vi "InterfaceExample.vi"() -> ()   [LabVIEW 2017]
uses:
  Interface/Configuration.ctl
  <instrlib>/_niInstr/FIFO Register Bus/v1/Host/niInstr FIFO Register Bus v1 Host.lvclass
  C:/Program Files (x86)/National Instruments/LabVIEW 2017/instr.lib/_niInstr/Instruction Framework/v1/Host/Instruction Target/niInstr Instruction Target v1 Host.lvclass
  <vilib>/FPGAPlugInAG/sbRIO-9607/niLvFpga_Open_sbRIO-9607.vi
  <vilib>/rvi/interface/common/dynamic/niFpgaDynamicAddResources.vi
  <vilib>/Utility/error.llb/Error Cluster From Error Code.vi
  <vilib>/rvi/errors/niLvFpgaAdjustHostInterfaceError.vi
  <vilib>/FPGAPlugInAG/Dynamic/niLvFpga_Close_Dynamic.vi
  <vilib>/rvi/interface/nirviOpenFPGA/nirviOpenFPGA.xnode
  FPGA Bitfiles/ScaleAndLimit_FPGATarget_BasicExampleWith_nkdyZl4UhlU.lvbitx
  <vilib>/rvi/interface/nirviReadWriteControl/nirviReadWriteControl.xnode
  <vilib>/rvi/interface/nirviCloseFPGA/nirviCloseFPGA.xnode
  Interface/ScaleAndLimitInterface.lvlib
  <instrlib>/_niInstr/Instruction Framework/v1/Host/Subsystem Map/niInstr Subsystem Map v1 Host.lvclass
  NiFpgaLv.dll
  <vilib>/rvi/interface/Simulation/niFpgaSimulationCallBeginRW.vi
panel:
  out "ScaledAI":sgl[](array[numeric])
  out "SimultaneousAILoopRate":u32
  in  "DummyChannel15":i16
  in  "stop":bool
  out "Limits":string
  in  "clearLimits":bool
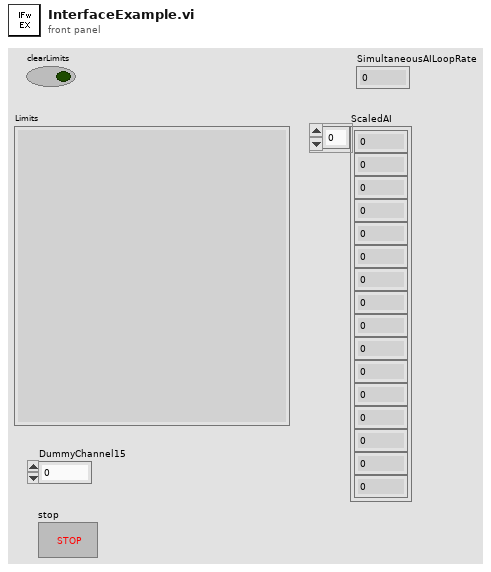
[diagram p1: front panel]
types:
  T1 = typedef "ScaleAndLimitInterface.lvlib/Configuration.ctl" = cluster{"Name":string, "M":dbl, "B":i16, "HighLimit":dbl, "LowLimit":dbl, "LimitsEnabled":bool}
  T2 = typedef "ScaleAndLimitInterface.lvlib/Interface.ctl" = cluster{"instruction target":refnum<class "niInstr Instruction Target v1 Host.lvclass">, "ScalingAndLimitsContext":refnum<class "niInstr Instruction Framework Context v1 Host.lvclass">, "Configuration":T1[]}
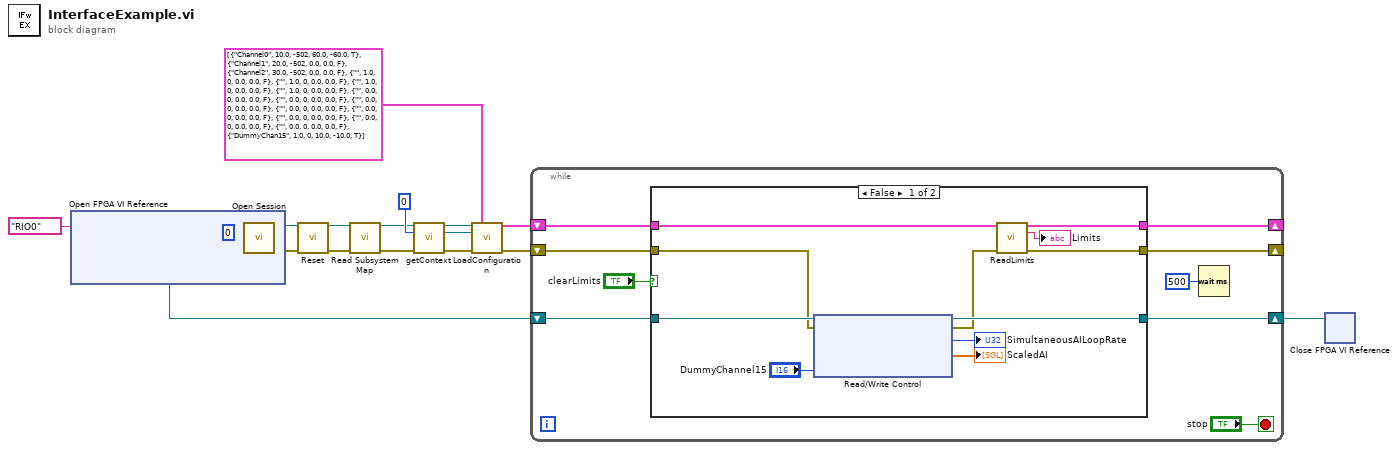
[diagram p0: block diagram]
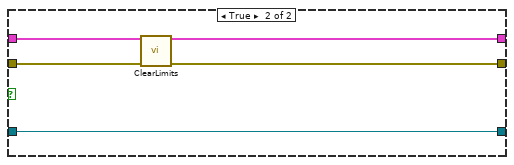
[diagram p2: hidden frame]
diagram:
  n1 = xnode "Open FPGA VI Reference"("resource name"=tag "RIO0") -> ("FPGA VI Reference Out"=w7:refnum<k20>, "error out"=w6:errorcluster)  [unwired: 1 in]
  n2 = call <instrlib>:"Open Session.vi"("fpga ref"=w7, "bus instance"=u32 0, "error in"=w6) -> ("session out"=w10:refnum<class "niInstr FIFO Register Bus v1 Host.lvclass">, "error out"=w11:errorcluster)  [unwired: 11 in]
  n3 = call-dynamic "Reset.vi"("session in"=w10, "error in"=w11) -> ("session out"=w8:refnum<class "niInstr FIFO Register Bus v1 Host.lvclass">, "error out"=w9:errorcluster)  [unwired: 12 in]
  n4 = call <instrlib>:"Read Subsystem Map.vi"("instruction target in"=w8, "error in"=w9) -> ("instruction target out"=w3:refnum<class "niInstr FIFO Register Bus v1 Host.lvclass">, "error out"=w5:errorcluster)  [unwired: 11 in, 1 out]
  n5 = call "getContext.vi"("session in"=w3, "instance"=u8 0, "error in"=w5) -> ("session out"=w2:refnum<class "niInstr FIFO Register Bus v1 Host.lvclass">, "ScalingAndLimitsContext"=w1:refnum<class "niInstr Instruction Framework Context v1 Host.lvclass">, "error out"=w17:errorcluster)  [unwired: 10 in]
  n6 = call "LoadConfiguration.vi"("instruction target in"=w2, "Configuration"=T1[] [{"Name"="Channel0", "M"=10.0, "B"=-502, "HighLimit"=60.0, "LowLimit"=-60.0, "LimitsEnabled"=TRUE}, {"Name"="Channel1", "M"=20.0, "B"=-502, "HighLimit"=0.0, "LowLimit"=0.0, "LimitsEnabled"=FALSE}, {"Name"="Channel2", "M"=30.0, "B"=-502, "HighLimit"=0.0, "LowLimit"=0.0, "LimitsEnabled"=FALSE}, {"Name"="", "M"=1.0, "B"=0, "HighLimit"=0.0, "LowLimit"=0.0, "LimitsEnabled"=FALSE}, {"Name"="", "M"=1.0, "B"=0, "HighLimit"=0.0, "LowLimit"=0.0, "LimitsEnabled"=FALSE}, {"Name"="", "M"=1.0, "B"=0, "HighLimit"=0.0, "LowLimit"=0.0, "LimitsEnabled"=FALSE}, {"Name"="", "M"=1.0, "B"=0, "HighLimit"=0.0, "LowLimit"=0.0, "LimitsEnabled"=FALSE}, {"Name"="", "M"=0.0, "B"=0, "HighLimit"=0.0, "LowLimit"=0.0, "LimitsEnabled"=FALSE}, {"Name"="", "M"=0.0, "B"=0, "HighLimit"=0.0, "LowLimit"=0.0, "LimitsEnabled"=FALSE}, {"Name"="", "M"=0.0, "B"=0, "HighLimit"=0.0, "LowLimit"=0.0, "LimitsEnabled"=FALSE}, {"Name"="", "M"=0.0, "B"=0, "HighLimit"=0.0, "LowLimit"=0.0, "LimitsEnabled"=FALSE}, {"Name"="", "M"=0.0, "B"=0, "HighLimit"=0.0, "LowLimit"=0.0, "LimitsEnabled"=FALSE}, {"Name"="", "M"=0.0, "B"=0, "HighLimit"=0.0, "LowLimit"=0.0, "LimitsEnabled"=FALSE}, {"Name"="", "M"=0.0, "B"=0, "HighLimit"=0.0, "LowLimit"=0.0, "LimitsEnabled"=FALSE}, {"Name"="", "M"=0.0, "B"=0, "HighLimit"=0.0, "LowLimit"=0.0, "LimitsEnabled"=FALSE}, {"Name"="DummyChan15", "M"=1.0, "B"=0, "HighLimit"=10.0, "LowLimit"=-10.0, "LimitsEnabled"=TRUE}], "ScalingAndLimitsContext"=w1, "error in (no error)"=w17) -> ("Interface"=w14:T2, "error out"=w13:errorcluster)  [unwired: 10 in]
  n7 = while {
    shift-right: [w20] -> _
    shift-left: w14 -> [w27]
    shift-right: [w19] -> _
    shift-left: w13 -> [w26]
    shift-right: [w21] -> w12
    shift-left: w7 -> [w22]
    stop <- "stop" stop-if-true
    n8 = case shown="False" "clearLimits" {
      tunnel: w27 -> [w34 w43]
      tunnel: w26 -> [w36 w42]
      tunnel: [w33 w41] -> w20
      tunnel: [w32 w40] -> w19
      tunnel: w22 -> [w38 w39]
      tunnel: [w35 w39] -> w21
      frame False {
        n9 = xnode "Read/Write Control"("FPGA VI Reference In"=w38, "error in"=w36, "DummyChannel15"="DummyChannel15") -> ("FPGA VI Reference Out"=w35:refnum<k20>, "error out"=w30:errorcluster, "SimultaneousAILoopRate"=→"SimultaneousAILoopRate":u32, "ScaledAI"=→"ScaledAI":sgl[])
        n10 = call "ReadLimits.vi"("Interface in"=w34, "error in (no error)"=w30) -> ("Interface out"=w33:T2, "Limits"=→"Limits":string, "error out"=w32:errorcluster)  [unwired: 11 in]
      }
      frame True {
        n11 = call "ClearLimits.vi"("Interface in"=w43, "error in (no error)"=w42) -> ("Interface out"=w41:T2, "error out"=w40:errorcluster)  [unwired: 12 in]
      }
    }
    n12 = Wait (ms)(milliseconds to wait=u32 500) -> ()  [unwired: 1 out]
  }
  n13 = xnode "Close FPGA VI Reference"("FPGA VI Reference In"=w12) -> ()  [unwired: 1 in, 1 out]
